vi "Separate Particles.vi"(11 "Objects":T1(array[cluster])) -> (0 "H Scores":T2(array[cluster]), 3 "V Scores":T2(array[cluster]))   [LabVIEW 2025]
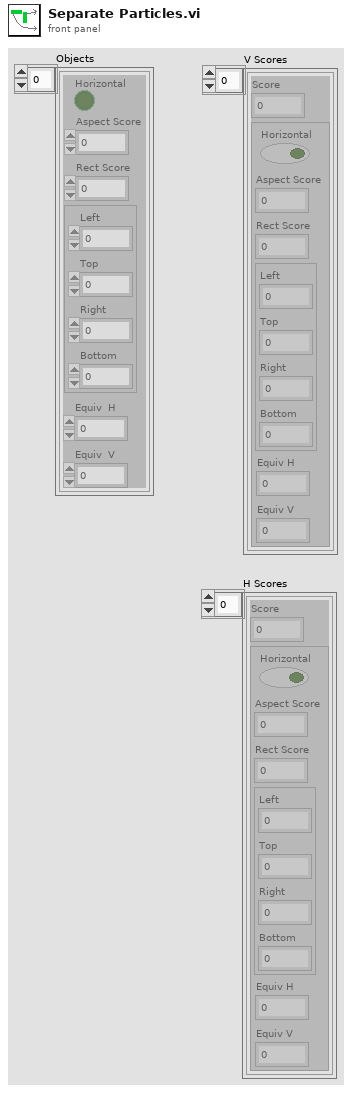
[diagram p1: front panel]
types:
  T1 = cluster{"Horizontal":bool, "Aspect Score":dbl, "Rect Score":dbl, cluster{"Left":dbl, "Top":dbl, "Right":dbl, "Bottom":dbl}, "Equiv  H":dbl, "Equiv  V":dbl}[]
  T2 = cluster{"Score":dbl, cluster{"Horizontal":bool, "Aspect Score":dbl, "Rect Score":dbl, cluster{"Left":dbl, "Top":dbl, "Right":dbl, "Bottom":dbl}, "Equiv H":dbl, "Equiv V":dbl}}[]
  T3 = cluster{"Score":dbl, cluster{"Horizontal":bool, "Aspect Score":dbl, "Rect Score":dbl, cluster{"Left":dbl, "Top":dbl, "Right":dbl, "Bottom":dbl}, "Long":dbl, "Short":dbl}}[]
  T4 = cluster{dbl, cluster{"Horizontal":bool, "Aspect Score":dbl, "Rect Score":dbl, cluster{"Left":dbl, "Top":dbl, "Right":dbl, "Bottom":dbl}, "Equiv  H":dbl, "Equiv  V":dbl}}
  T5 = cluster{"Score":dbl, cluster{"Horizontal":bool, "Aspect Score":dbl, "Rect Score":dbl, cluster{"Left":dbl, "Top":dbl, "Right":dbl, "Bottom":dbl}, "Equiv  H":dbl, "Equiv  V":dbl}}[]
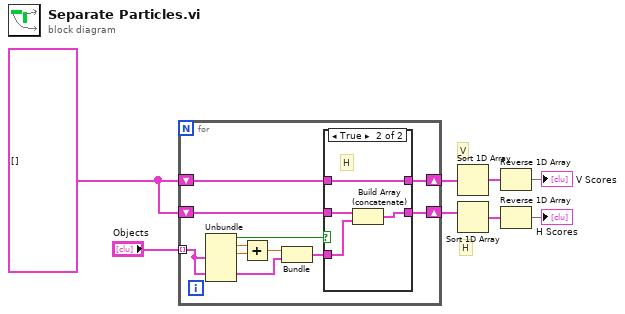
[diagram p0: block diagram]
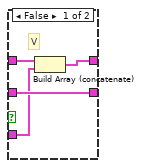
[diagram p2: hidden frame]
diagram:
  w1 = T3 [] ("V Scores")
  # "H"
  # "V"
  n1 = for {
    tunnel: "Objects" -> [w10] mode=indexing
    shift-right: [w14] -> w4
    shift-left: w1 -> [w15]
    shift-right: [w16] -> w3
    shift-left: w1 -> [w17]
    n2 = Unbundle(w10) -> ("Horizontal"=w18:bool, "Aspect Score"=w13:dbl, "Rect Score"=w12:dbl)  [unwired: 3 out]
    n3 = Add(x=w13, y=w12) -> (x+y=w11:dbl)
    n4 = Bundle(w11, w10) -> (w9:T4)  [unwired: 1 in]
    n5 = case shown="True" w18 {
      tunnel: w17 -> [w20 w26]
      tunnel: [w20 w25] -> w16
      tunnel: w15 -> [w22 w24]
      tunnel: [w21 w24] -> w14
      tunnel: w9 -> [w19 w23]
      frame False {
        # "V"
        n6 = Build Array (concatenate)(w22, w19) -> (w21:T5)
      }
      frame True {
        # "H"
        n7 = Build Array (concatenate)(w26, w23) -> (w25:T5)
      }
    }
  }
  n8 = Sort 1D Array(array=w4) -> (sorted array=w5:T3)
  n9 = Sort 1D Array(array=w3) -> (sorted array=w6:T3)
  n10 = Reverse 1D Array(array=w5) -> (reversed array=→"V Scores":T3)
  n11 = Reverse 1D Array(array=w6) -> (reversed array=→"H Scores":T3)
